vi "Read Initialize Command.vi"   [LabVIEW 2023, in "Cycler.lvclass"]
uses:
  Cycler.lvclass
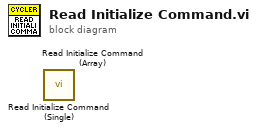
[diagram p0: block diagram]
diagram:
  n1 = call "Read Initialize Command (Single).vi"() -> ()  [unwired: 8 in, 4 out]
  n2 = call "Read Initialize Command (Array).vi"() -> ()  [unwired: 8 in, 4 out]
